vi "globalTearDown.vi"(8 "error in":errorcluster, 11 "Loopback in":refnum<class "Logging Loopback.lvclass">) -> (0 "error out":errorcluster, 3 "Loopback out":refnum<class "Logging Loopback.lvclass">)   [LabVIEW 2020, in "Logging Loopback.lvclass"]
uses:
  Logging Loopback.lvclass
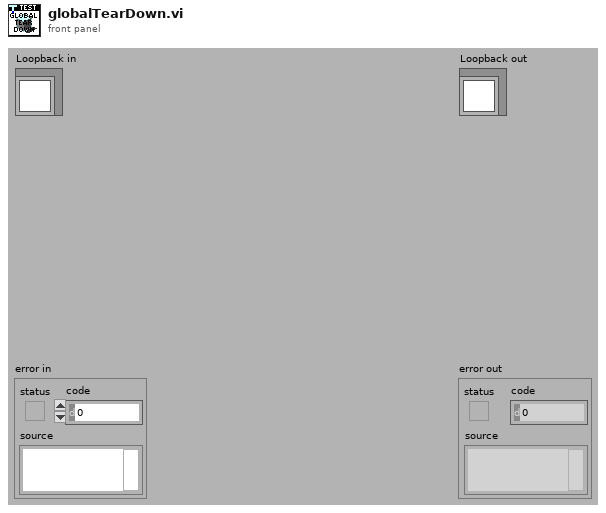
[diagram p1: front panel]
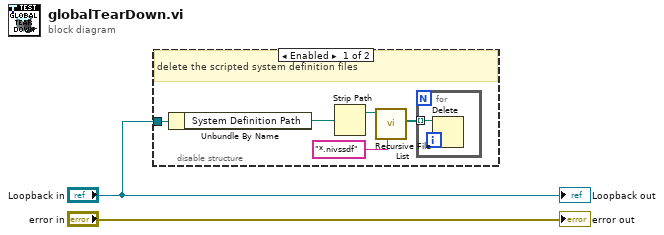
[diagram p0: block diagram]
diagram:
  n1 = disable-structure shown="Enabled" {
    disable-tunnel: "Loopback in" -> [w7 _]
    frame Enabled {
      # "delete the scripted system definition files"
      n2 = Unbundle By Name(w7) -> ("System Definition Path"=w4:path)
      n3 = Strip Path(path=w4) -> (stripped path=w3:path)  [unwired: 1 out]
      n4 = call <vilib>:"Recursive File List.vi"("pattern"="*.nivssdf", "Folder Path"=w3) -> ("All Files in Dir"=w5:path[])  [unwired: 5 in, 4 out]
      n5 = for {
        tunnel: w5 -> [w8] mode=indexing
        n6 = Delete(path (use dialog)=w8) -> ()  [unwired: 4 in, 3 out]
      }
    }
    frame Disabled {
    }
  }
  "error out" <- "error in"
  "Loopback out" <- "Loopback in"
